vi "Write Strings.vi"(8 "error in (no error)":errorcluster, 10 "Strings":string[](array[string]), 11 "Ring D Element in":refnum<class "String dropdown D Element.lvclass">) -> (0 "error out":errorcluster, 3 "Ring D Element out":refnum<class "String dropdown D Element.lvclass">)   [LabVIEW 2018, in "D Datagrid Library.lvlib" / "String dropdown D Element.lvclass"]
uses:
  String dropdown D Element.lvclass
  String dropdown D Element.lvclass/String dropdown D Element.ctl
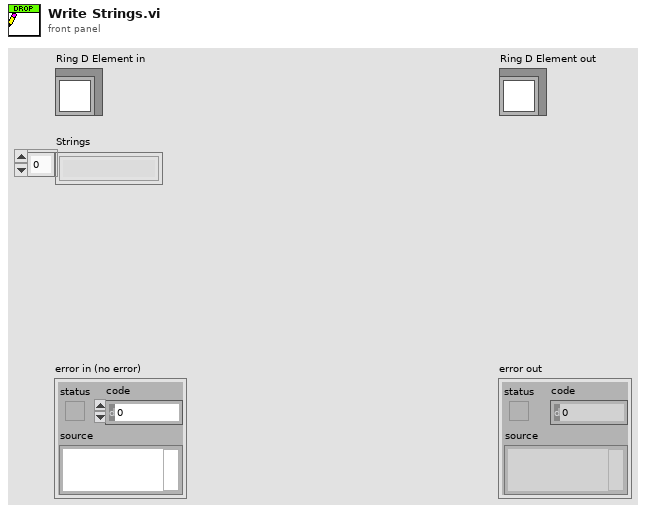
[diagram p1: front panel]
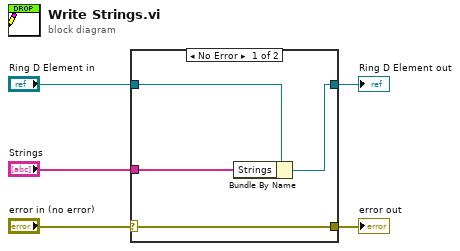
[diagram p0: block diagram]
diagram:
  n1 = case shown="No Error" "error in (no error)" {
    selector: "error in (no error)" -> [w9 w10]
    tunnel: [w9 w10] -> w4
    tunnel: [w7 w11] -> w2
    tunnel: "Ring D Element in" -> [w8 w11]
    tunnel: "Strings" -> [w6 _]
    frame No Error {
      n2 = Bundle By Name(cluster=w8, "Strings"=w6) -> (w7:refnum<class "String dropdown D Element.lvclass">)
    }
    frame Error {
    }
  }
  "error out" <- w4
  "Ring D Element out" <- w2
